vi "Read_ini_ArraySection.vi"(8 "error in (no error)":errorcluster, 10 "ArraySection":string[](array[string]), 11 "configuration file path":path) -> (0 "error out":errorcluster, 2 "ArrayValue":dbl[][](array[numeric]))   [LabVIEW 2015]
uses:
  <vilib>/Utility/config.llb/Read Key (String).vi
  <vilib>/Utility/config.llb/NI_LVConfig.lvlib
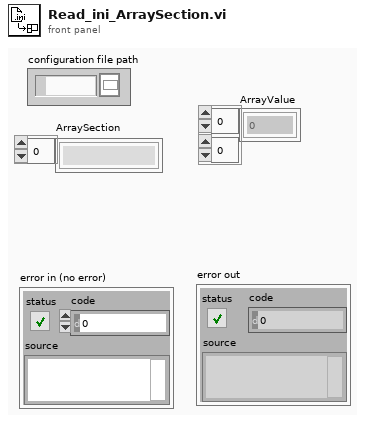
[diagram p1: front panel]
types:
  T1 = typedef "NI_LVConfig.lvlib/Config Data RefNum.ctl" = refnum<k1>
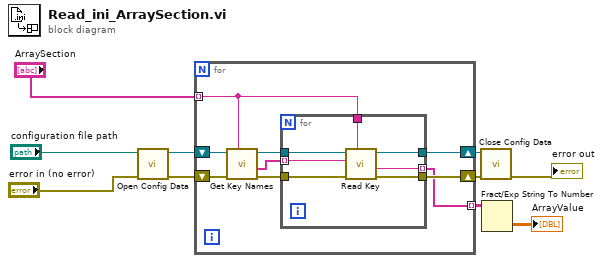
[diagram p0: block diagram]
diagram:
  n1 = call <vilib>:"Open Config Data.vi"("error in (no error)"="error in (no error)", "configuration file path"="configuration file path") -> ("error out"=w5:errorcluster, "refnum"=w4:T1)  [unwired: 7 in, 1 out]
  n2 = for {
    tunnel: [w12] -> w3 mode=indexing
    tunnel: "ArraySection" -> [w11] mode=indexing
    shift-right: [w19] -> w9
    shift-left: w5 -> [w17]
    shift-right: [w18] -> w8
    shift-left: w4 -> [w16]
    n3 = call <vilib>:"Get Key Names.vi"("section"=w11, "error in (no error)"=w17, "refnum"=w16) -> ("error out"=w14:errorcluster, "key names"=w13:string[], "refnum out"=w15:T1)  [unwired: 5 in, 1 out]
    n4 = for {
      tunnel: [w26] -> w19
      tunnel: [w25] -> w18
      tunnel: w11 -> [w24]
      tunnel: w15 -> [w23]
      tunnel: w14 -> [w22]
      tunnel: w13 -> [w21] mode=indexing
      tunnel: [w20] -> w12 mode=indexing
      n5 = call-poly <vilib>:"Read Key.vi"("section"=w24, "error in (no error)"=w22, "key"=w21, "refnum"=w23) -> ("error out"=w26:errorcluster, "value"=w20:string, "refnum out"=w25:T1)  [unwired: 4 in, 1 out]
    }
  }
  n6 = call <vilib>:"Close Config Data.vi"("error in (no error)"=w9, "refnum"=w8) -> ("error out"=→"error out":errorcluster)  [unwired: 8 in, 1 out]
  n7 = Fract/Exp String To Number(string=w3) -> (number=→"ArrayValue":dbl[][])  [unwired: 3 in, 1 out]
